vi "Read URL Encoded Form.vi"(8 "error in (no error)":errorcluster, 9 "Stream in":refnum<k5>, 11 "Request in":refnum<class "Request.lvclass">) -> (0 "error out":errorcluster, 1 "Stream out":refnum<k5>, 3 "Request out":refnum<class "Request.lvclass">)   [LabVIEW 2020, in "HTTP Utils.lvlib" / "Request.lvclass"]
uses:
  Request.lvclass
  Request.lvclass/Request.ctl
  FormField/FormField.lvclass
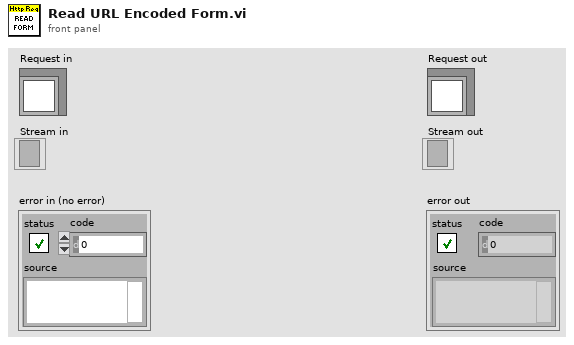
[diagram p1: front panel]
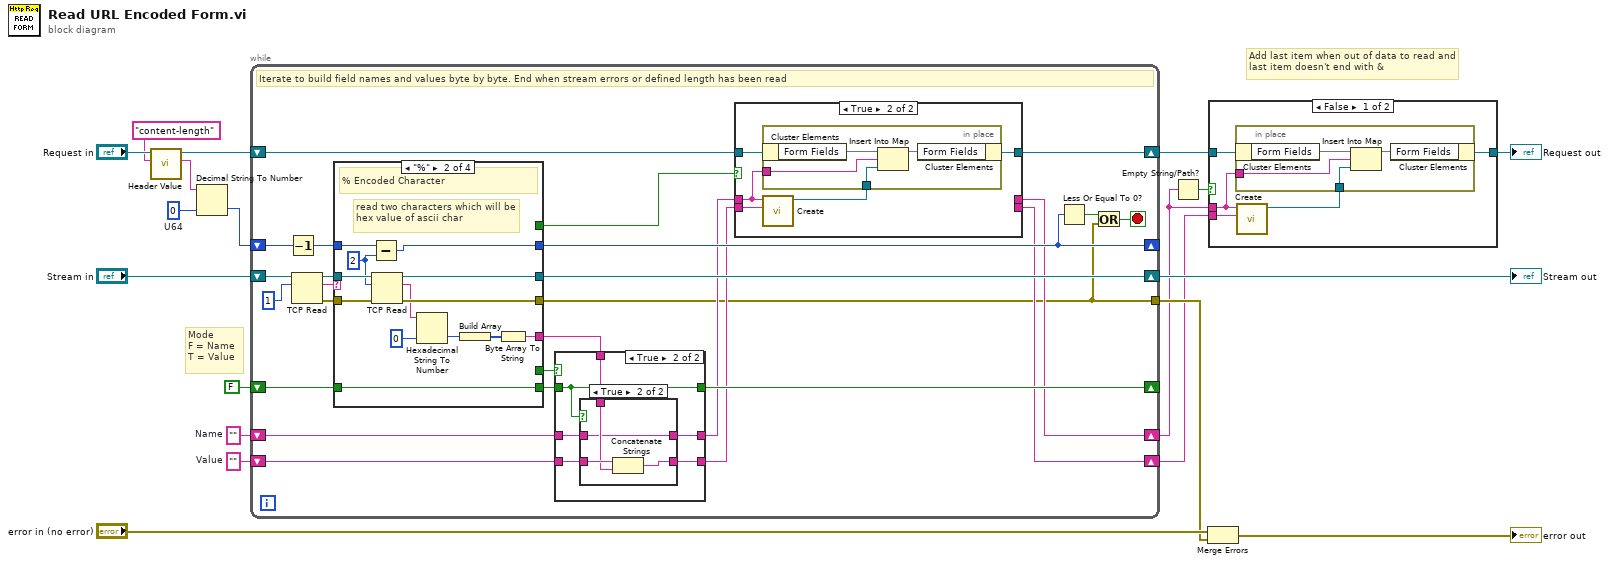
[diagram p0: block diagram]
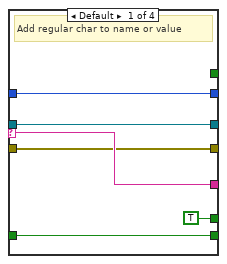
[diagram p2: hidden frame]
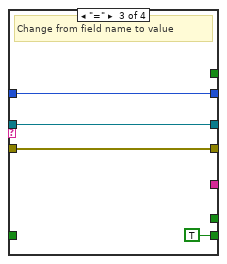
[diagram p3: hidden frame]
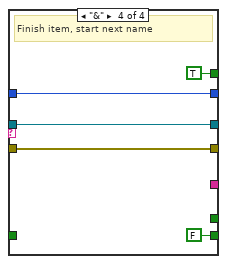
[diagram p4: hidden frame]
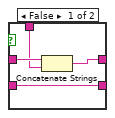
[diagram p6: hidden frame]
diagram:
  w5 = ""  # Value
  w7 = ""  # Name
  w11 = u64 0  # U64
  # "Add last item when out of data to read and last item doesn't end with &"
  # "Mode\nF = Name\nT = Value"
  n1 = call "Header Value.vi"("Header"="content-length", "Request in"="Request in") -> ("Value"=w12:string, "Request out"=w8:refnum<class "Request.lvclass">)  [unwired: 6 in, 2 out]
  n2 = Decimal String To Number(string=w12, default (0L)=w11) -> (number=w9:u64)  [unwired: 1 in, 1 out]
  n3 = while {
    shift-right: [w22] -> w4
    shift-left: w8 -> [w33]
    shift-right: [w37] -> w14
    shift-left: "Stream in" -> [w45]
    shift-right: [w24] -> w2
    shift-left: w7 -> [w28]
    shift-right: [w39] -> _
    shift-left: w9 -> [w43]
    shift-right: [w30] -> _
    shift-left: FALSE -> [w35]
    shift-right: [w23] -> w1
    shift-left: w5 -> [w27]
    tunnel: [w20] -> w16
    stop <- w21 stop-if-true
    # "Iterate to build field names and values byte by byte. End when stream errors or defined length has been read"
    n4 = Decrement(x=w43) -> (x-1=w41:u64)
    n5 = TCP Read(connection ID=w45, bytes to read=1 ("Count")) -> (connection ID out=w40:refnum<k5>, data out=w38:string, error out=w36:errorcluster)  [unwired: 3 in]
    n6 = case shown="\"%\"" w38 {
      selector: w38 -> [w50 _ _ _]
      tunnel: w41 -> [w48 w63 w67 w70]
      tunnel: w40 -> [w51 w64 w66 w73]
      tunnel: [w48 w61 w67 w70] -> w39
      tunnel: [w51 w59 w66 w73] -> w37
      tunnel: [w50 w56 _ _] -> w29
      tunnel: w36 -> [w49 w55 w65 w72]
      tunnel: [w49 w54 w65 w72] -> w20
      tunnel: w35 -> [w47 w52 _ _]
      tunnel: [w47 w52 TRUE FALSE] -> w34
      tunnel: [_ _ _ TRUE] -> w32
      tunnel: [TRUE _ _ _] -> w31
      frame Default {
        # "Add regular char to name or value"
      }
      frame "%" {
        w62 = 2 ("Count")
        # "read two characters which will be hex value of ascii char"
        # "% Encoded Character"
        n7 = Subtract(x=w63, y=w62) -> (x-y=w61:u64)
        n8 = TCP Read(connection ID=w64, bytes to read=w62, error in (no error)=w55) -> (connection ID out=w59:refnum<k5>, data out=w53:string, error out=w54:errorcluster)  [unwired: 2 in]
        n9 = Hexadecimal String To Number(string=w53, default (0uL)=u8 0 ("default (0 U32)")) -> (number=w58:u8)  [unwired: 1 in, 1 out]
        n10 = Build Array(w58) -> (w57:u8[])
        n11 = Byte Array To String(unsigned byte array=w57) -> (string=w56:string)
      }
      frame "=" {
        # "Change from field name to value"
      }
      frame "&" {
        # "Finish item, start next name"
      }
    }
    n12 = case shown="True" w31 {
      tunnel: w34 -> [w74 w82]
      tunnel: w28 -> [w76 w81]
      tunnel: [w76 w77] -> w26
      tunnel: [w75 w78] -> w25
      tunnel: w27 -> [w75 w80]
      tunnel: [w74 w82] -> w30
      tunnel: w29 -> [_ w79]
      frame False {
      }
      frame True {
        n13 = case shown="True" w82 {
          tunnel: w81 -> [w86 w87]
          tunnel: w80 -> [w84 w90]
          tunnel: w79 -> [w85 w89]
          tunnel: [w84 w88] -> w78
          tunnel: [w83 w87] -> w77
          frame False {
            n14 = Concatenate Strings(w86, w85) -> (w83:string)
          }
          frame True {
            n15 = Concatenate Strings(w90, w89) -> (w88:string)
          }
        }
      }
    }
    n16 = case shown="True" w32 {
      tunnel: w33 -> [w91 w97]
      tunnel: w26 -> [w93 w95]
      tunnel: w25 -> [w92 w98]
      tunnel: [w93 _] -> w24
      tunnel: [w92 _] -> w23
      tunnel: [w91 w94] -> w22
      frame False {
      }
      frame True {
        n17 = call "Create.vi"("Value"=w98, "Name"=w95) -> ("FormField"=w96:refnum<class "FormField.lvclass">)  [unwired: 9 in]
        n18 = in-place {
          in-place-border: w96 -> [w100]
          in-place-border: w95 -> [w101]
          n19 = in-place-cluster #1(w97) -> ("Form Fields"=w102:map{string, refnum<class "FormField.lvclass">})
          n20 = Insert Into Map(map in=w102, key=w101, value=w100) -> (map out=w99:map{string, refnum<class "FormField.lvclass">})  [unwired: 2 out]
          n21 = in-place-cluster #1("Form Fields"=w99) -> (w94:refnum<class "Request.lvclass">)
        }
      }
    }
    n22 = Less Or Equal To 0?(x=w39) -> (x <= 0?=w42:bool)
    n23 = Or(x=w42, y=w20) -> (x .or. y?=w21:bool)
  }
  "Stream out" <- w14
  n24 = Empty String/Path?(string/path=w2) -> (empty?=w3:bool)
  n25 = Merge Errors("error in (no error)", w16) -> (→"error out":errorcluster)
  n26 = case shown="False" w3 {
    tunnel: w4 -> [w106 w112]
    tunnel: w2 -> [w104 _]
    tunnel: w1 -> [w107 _]
    tunnel: [w103 w112] -> w18
    frame False {
      n27 = call "Create.vi"("Value"=w107, "Name"=w104) -> ("FormField"=w105:refnum<class "FormField.lvclass">)  [unwired: 9 in]
      n28 = in-place {
        in-place-border: w105 -> [w109]
        in-place-border: w104 -> [w110]
        n29 = in-place-cluster #2(w106) -> ("Form Fields"=w111:map{string, refnum<class "FormField.lvclass">})
        n30 = Insert Into Map(map in=w111, key=w110, value=w109) -> (map out=w108:map{string, refnum<class "FormField.lvclass">})  [unwired: 2 out]
        n31 = in-place-cluster #2("Form Fields"=w108) -> (w103:refnum<class "Request.lvclass">)
      }
    }
    frame True {
    }
  }
  "Request out" <- w18
